vi "Initialise Tab Control.vi"(8 "error in":errorcluster, 11 "Tab Control Reference In":refnum<vi>) -> (0 "error out":errorcluster)   [LabVIEW 2017, in "DTacq Plot Display Library.lvlib"]
doc: "Prepares the graphical user interface for display;\nGUI controls are set to their default values,\nThe front panel is centered on the screen,\nThe front panel is opened, if not already open"
uses:
  DTacq Plot Display Library.lvlib
panel:
  out "Tab Control Reference Out":refnum<vi>
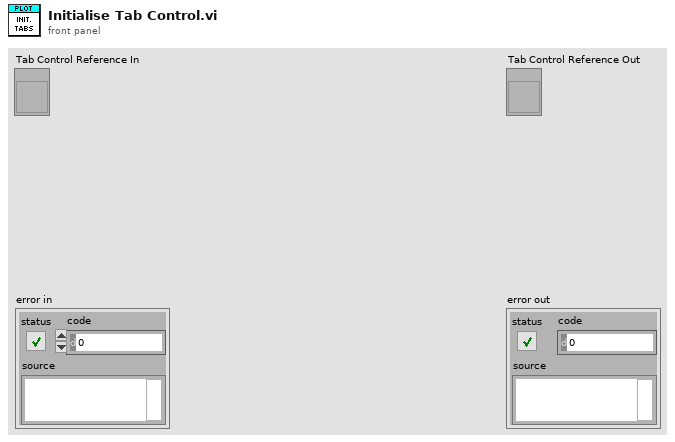
[diagram p1: front panel]
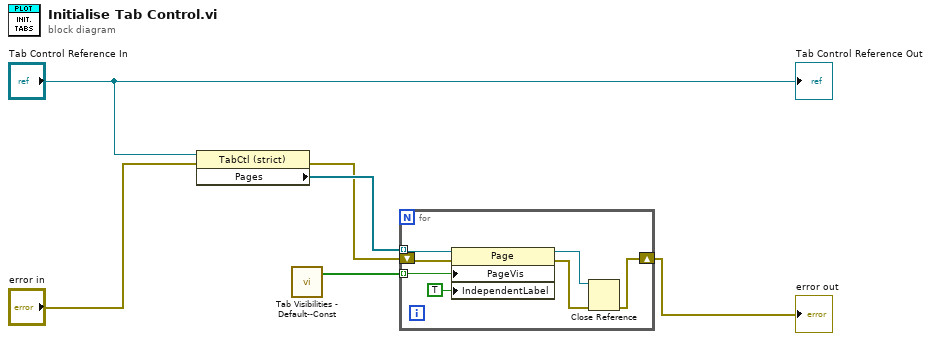
[diagram p0: block diagram]
diagram:
  n1 = property class="TabCtl (strict)"(reference="Tab Control Reference In", error in="error in") -> (error out=w2:errorcluster, "Pages"=w3:refnum<vi>[])  [unwired: 1 out]
  n2 = call "Tab Visibilities - Default--Const.vi"() -> ("Tab Visbility"=w4:bool[])  [unwired: 11 in]
  n3 = for {
    tunnel: w4 -> [w10] mode=indexing
    tunnel: w3 -> [w13] mode=indexing
    shift-right: [w9] -> w1
    shift-left: w2 -> [w12]
    n4 = property class="Page"(reference=w13, error in=w12, "PageVis"=w10, "IndependentLabel"=TRUE ("Independent Label")) -> (reference out=w8:refnum<vi>, error out=w11:errorcluster)
    n5 = Close Reference(reference=w8, error in (no error)=w11) -> (error out=w9:errorcluster)
  }
  "error out" <- w1
  "Tab Control Reference Out" <- "Tab Control Reference In"
